vi "loadHEXAFile1.vi"(7 "working directory":path=path "c:/temp", 11 "Path":string) -> ()   [LabVIEW 2012]
uses:
  <vilib>/addons/database/Connection.llb/DB Tools Open Connec (Path).vi
  <vilib>/addons/database/Connection.llb/Conn Execute.vi
  <vilib>/addons/database/Recordset.llb/Rec Fetch Recordset Data (R).vi
  <vilib>/addons/database/Recordset.llb/Rec Destroy - Connection.vi
  <vilib>/addons/database/_DB Variant To Data/Database Variant To Data.xnode
  <vilib>/addons/database/NI_Database_API.lvlib
panel:
  out "concatenated string":string
  out "error out":errorcluster
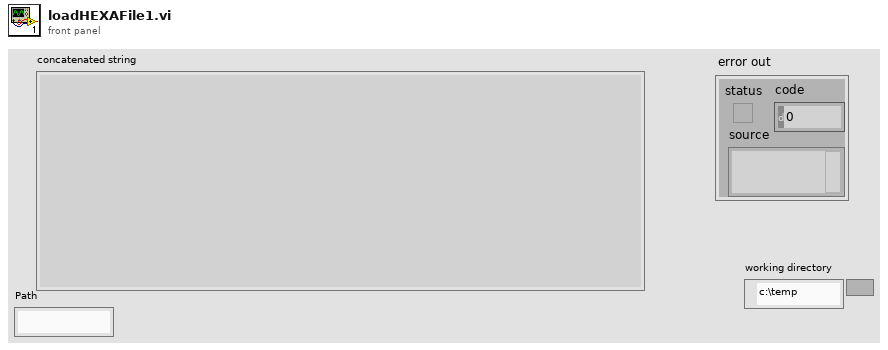
[diagram p1: front panel]
types:
  T1 = typedef "NI_Database_API.lvlib/Conn ObjectReference.ctl" = refnum<k1>
  T2 = typedef "NI_Database_API.lvlib/Rec ObjectReference.ctl" = refnum<k1>
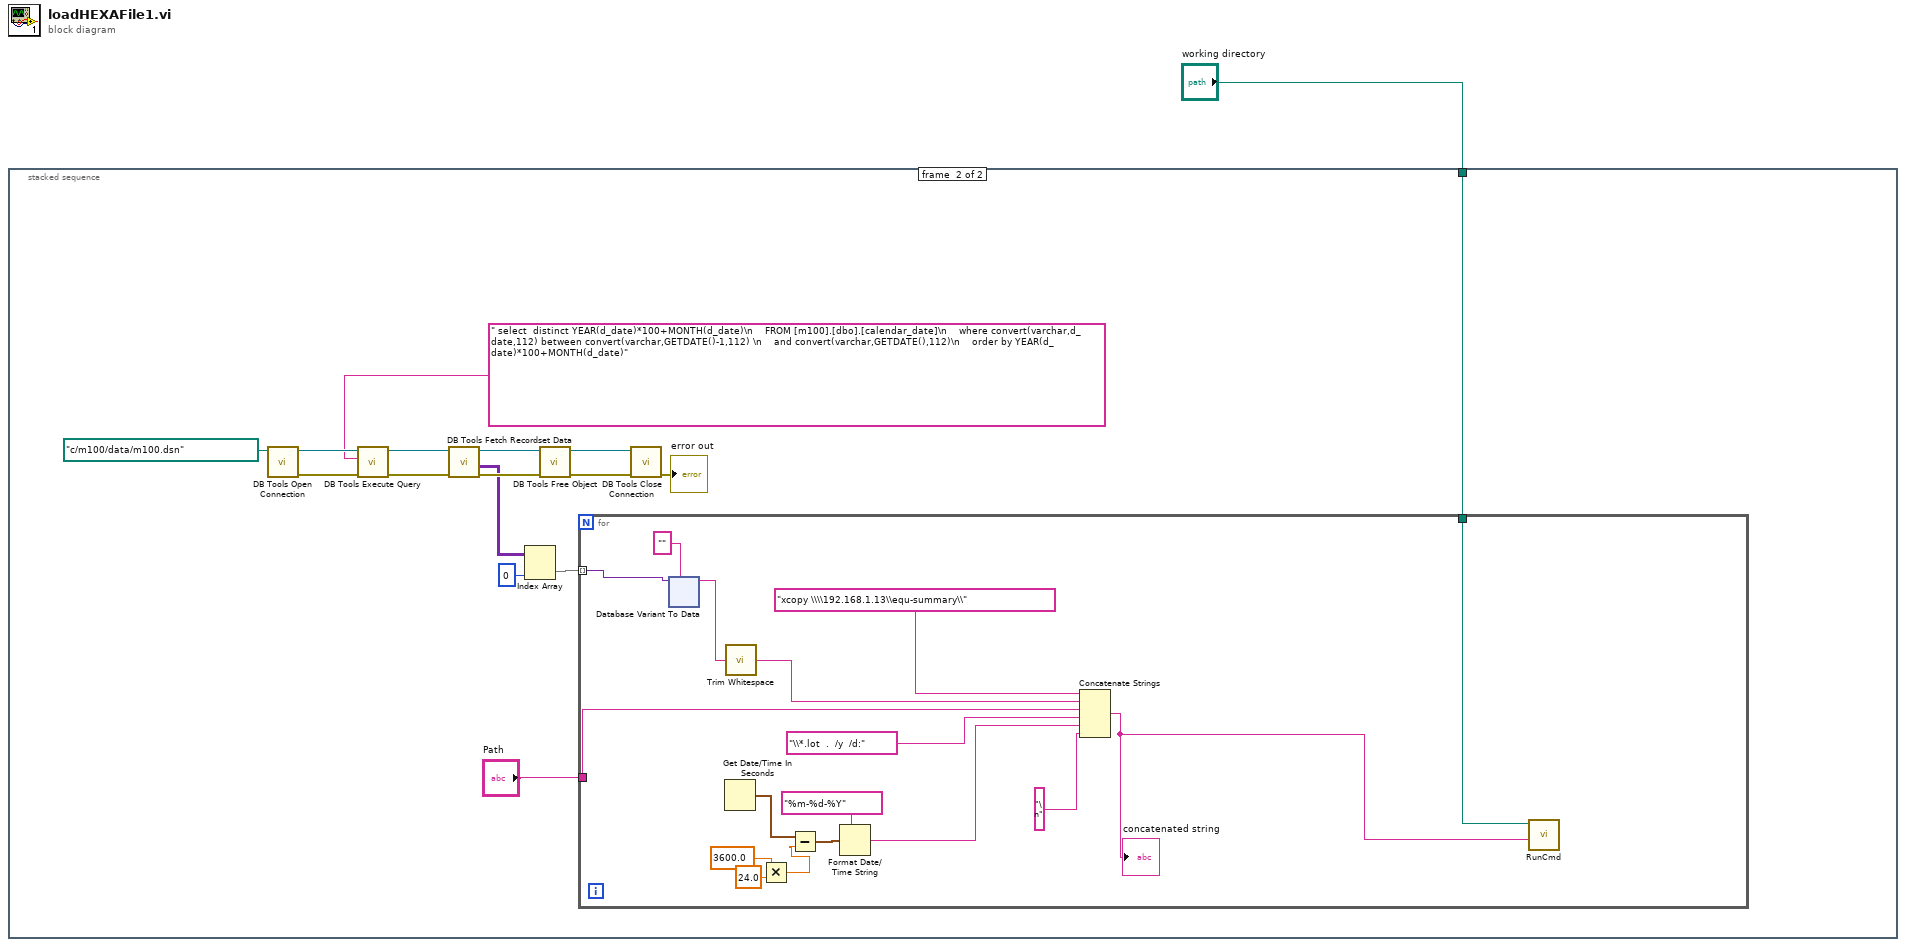
[diagram p0: block diagram]
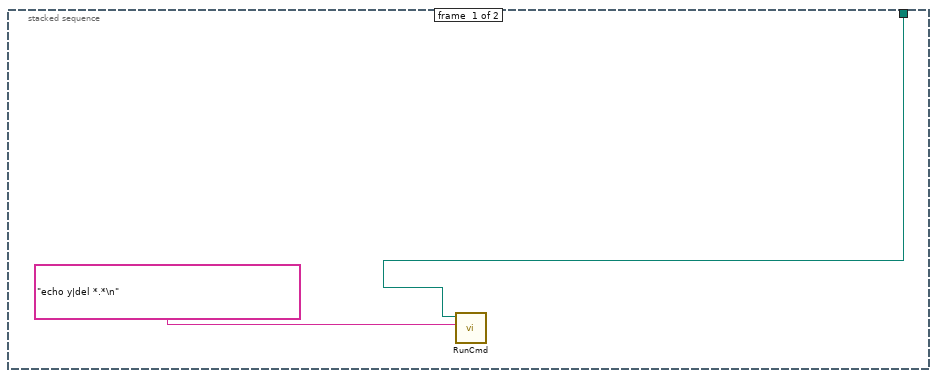
[diagram p2: hidden frame]
diagram:
  n1 = stacked-sequence {
    tunnel: "working directory" -> [w2 w4]
    frame #0 {
      n2 = call "RunCmd.vi"("Cmd String"="echo y|del *.*\n" ("standard input"), "working directory"=w2) -> ()  [unwired: 8 in, 2 out]
    }
    frame #1 {
      n3 = call-poly <vilib>:"DB Tools Open Connection.vi"("connection information"=path "c:/m100/data/m100.dsn") -> ("error out"=w15:errorcluster, "connection reference"=w19:T1)  [unwired: 7 in]
      n4 = call-poly <vilib>:"DB Tools Execute Query.vi"("error in (no error)"=w15, "SQL query"=" select  distinct YEAR(d_date)*100+MONTH(d_date)\n    FROM [m100].[dbo].[calendar_date]\n    where convert(varchar,d_date,112) between convert(varchar,GETDATE()-1,112) \n    and convert(varchar,GETDATE(),112)\n    order by YEAR(d_date)*100+MONTH(d_date)", "connection reference"=w19) -> ("error out"=w14:errorcluster, "recordset reference"=w18:T2)  [unwired: 5 in]
      n5 = call-poly <vilib>:"DB Tools Fetch Recordset Data.vi"("error in (no error)"=w14, "recordset reference"=w18) -> ("error out"=w13:errorcluster, "recordset data"=w8:variant[][], "recordset reference out"=w17:T2)  [unwired: 3 in]
      n6 = Index Array(array=w8, index (col)=0 ("disabled index (col)")) -> (element=w6:variant[])  [unwired: 1 in]
      n7 = call-poly <vilib>:"DB Tools Free Object.vi"("error in (no error)"=w13, "recordset reference"=w17) -> ("error out"=w12:errorcluster, "connection reference"=w16:T1)  [unwired: 8 in]
      n8 = for {
        tunnel: w6 -> [w36] mode=indexing
        tunnel: "Path" -> [w22]
        tunnel: w4 -> [w20]
        n9 = xnode "Database Variant To Data"("database variant"=w36, "type"="") -> ("data"=w26:string)  [unwired: 1 in, 1 out]
        n10 = Get Date/Time In Seconds() -> (seconds since 1Jan1904=w27:timestamp)
        n11 = call <vilib>:"Trim Whitespace.vi"("string"=w26) -> ("trimmed string"=w23:string)  [unwired: 1 in]
        n12 = Multiply(x=3600.0, y=24.0) -> (x*y=w29:dbl)
        n13 = Subtract(x=w27, y=w29) -> (x-y=w30:timestamp)
        n14 = Format Date/Time String(time format string (%c)="%m-%d-%Y", seconds (now)=w30) -> (date/time string=w32:string)  [unwired: 1 in]
        n15 = Concatenate Strings("xcopy \\\\192.168.1.13\\equ-summary\\" ("string"), w23, w22, "\\*.lot  .  /y  /d:" ("string"), w32, "\n" ("string")) -> (w21:string)
        "concatenated string" <- w21
        n16 = call "RunCmd.vi"("Cmd String"=w21, "working directory"=w20) -> ()  [unwired: 8 in, 2 out]
      }
      n17 = call <vilib>:"DB Tools Close Connection.vi"("error in (no error)"=w12, "connection reference"=w16) -> ("error out"=→"error out":errorcluster)  [unwired: 5 in]
    }
  }
